vi "to string 1.0.vi"(8 "error in (no error)":errorcluster, 11 "ResultProcessor Config in":refnum<class "ResultProcessor Config.lvclass">) -> (0 "error out":errorcluster, 2 "data":string, 3 "ResultProcessor Config out":refnum<class "ResultProcessor Config.lvclass">)   [LabVIEW 2015, in "ResultProcessor Config.lvclass"]
uses:
  ResultProcessor Config.lvclass
  ResultProcessor Config.lvclass/ResultProcessor Config.ctl
  <vilib>/NI/Configuration Framework/serializable configuration/NISE_CEF_serializable configuration.lvclass
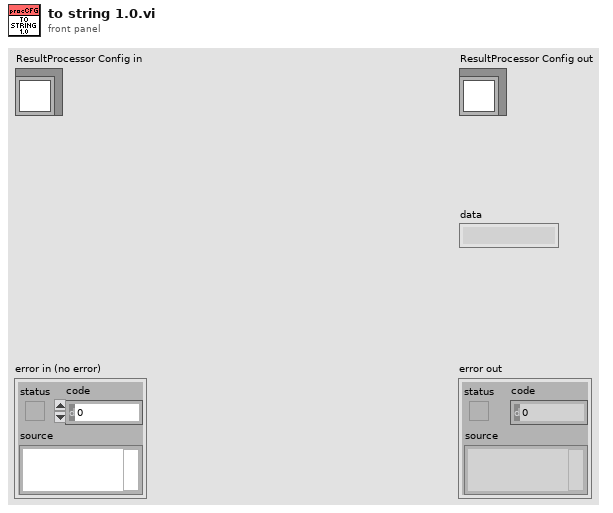
[diagram p1: front panel]
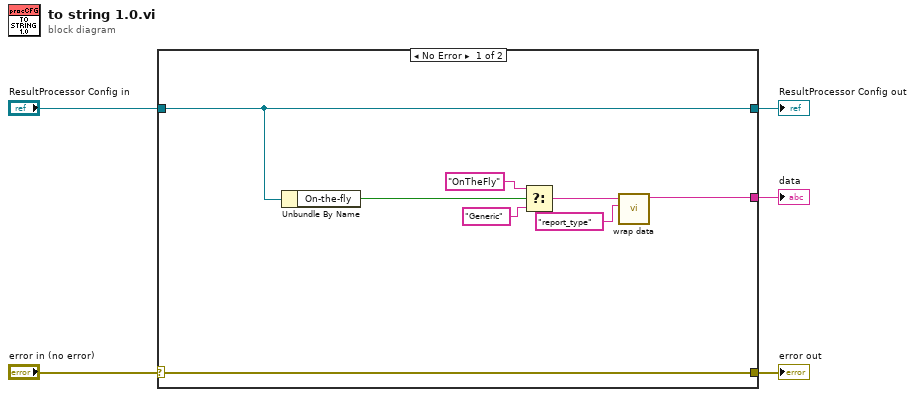
[diagram p0: block diagram]
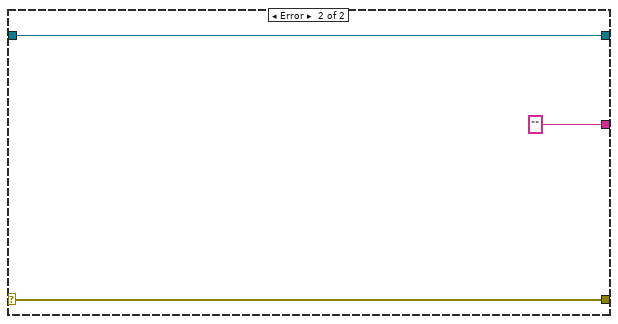
[diagram p2: hidden frame]
diagram:
  n1 = case shown="No Error" "error in (no error)" {
    selector: "error in (no error)" -> [w13 w16]
    tunnel: [w13 w16] -> w4
    tunnel: [w7 w15] -> w2
    tunnel: "ResultProcessor Config in" -> [w7 w15]
    tunnel: [w8 ""] -> w1
    frame No Error {
      n2 = Unbundle By Name(w7) -> ("On-the-fly"=w6:bool)
      n3 = Select(t="OnTheFly" ("identifier"), s=w6, f="Generic" ("identifier")) -> (s? t:f=w12:string)
      n4 = call <vilib>:"wrap data.vi"("identifier"="report_type", "data to wrap"=w12) -> ("wrapped data"=w8:string)  [unwired: 9 in]
    }
    frame Error {
    }
  }
  "error out" <- w4
  "ResultProcessor Config out" <- w2
  "data" <- w1
